vi "API_Goto Cleaning Position.vi"(8 "error in (no error)":errorcluster) -> (0 "error out":errorcluster)   [LabVIEW 2015, in "Tool Module.lvlib"]
doc: "Moves the tool to the cleaning position (stored in the tool coniguration). After tool is at the cleaning position (stopped moving), return with API_GOTO.vi pos 0 or use the API_Init Home Position.vi"
uses:
  Tool Module.lvlib
  Support/_GoTo Cmd Typedef--enum.ctl
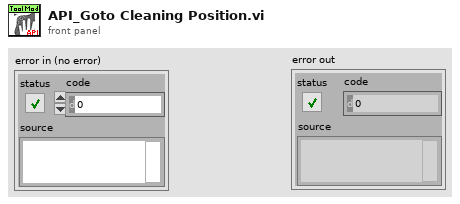
[diagram p1: front panel]
types:
  T1 = typedef "Tool Module.lvlib/_GoTo Cmd Typedef--enum.ctl" = enum16{"MoveA", "MoveR", "Home Position", "Home None", "Cleaning Position"}
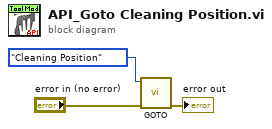
[diagram p0: block diagram]
diagram:
  n1 = call "GOTO.vi"("error in (no error)"="error in (no error)", "GoTo Cmd"=_GoTo_Cmd_Typedef--enum."Cleaning Position" ("_GoTo Cmd typedef")) -> ("error out"=→"error out":errorcluster)  [unwired: 9 in]
